vi "Data_to_refnum.vi"(7 "refnum in":T1, 8 "error in (no error)":errorcluster, 11 "DAQ refnum in":refnum<visa-resource-name>) -> (0 "error out":errorcluster, 3 "refnum out":T1)   [LabVIEW 2021, in "Korad KA3305P.lvlib"]
uses:
  Korad KA3305P.lvlib
  Reference.ctl
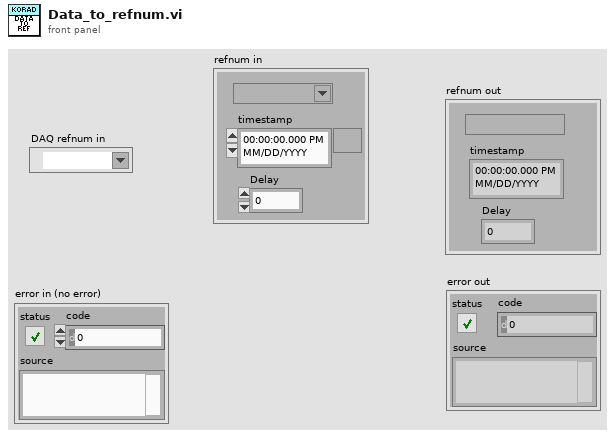
[diagram p1: front panel]
types:
  T1 = typedef "Korad KA3305P.lvlib/Reference.ctl" = cluster{"refnum":refnum<visa-resource-name>, "timestamp":timestamp, "Delay":dbl}
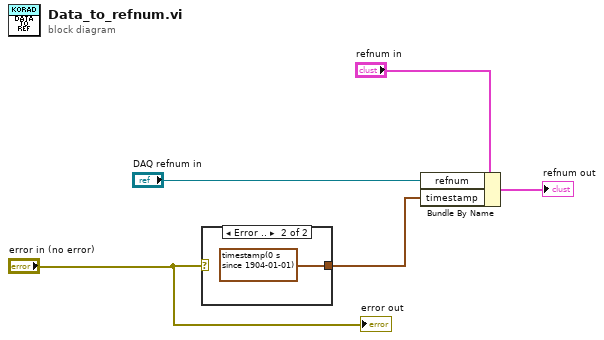
[diagram p0: block diagram]
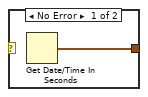
[diagram p2: hidden frame]
diagram:
  n1 = case shown="Error .." "error in (no error)" {
    tunnel: [w6 timestamp(0 s since 1904-01-01) ("seconds since 1Jan1904")] -> w5
    frame No Error {
      n2 = Get Date/Time In Seconds() -> (seconds since 1Jan1904=w6:timestamp)
    }
    frame Error {
    }
  }
  n3 = Bundle By Name(cluster="refnum in", "refnum"="DAQ refnum in", "timestamp"=w5) -> (→"refnum out":T1)
  "error out" <- "error in (no error)"
